vi "ESN_network.vi"(7 "In train phase? (F)":bool, 8 "error in (no error)":errorcluster, 9 "Desired output":dbl[](array[numeric]), 10 "input":dbl[](array[numeric]), 11 "ESN Status":T1) -> (0 "error out":errorcluster, 1 "State collection":dbl[](array[numeric]), 2 "output":dbl[](array[numeric]), 3 "ESN dup":T1)   [LabVIEW 2017]
uses:
  ESN_Network.ctl
  <vilib>/Analysis/Matrix/Datatypes/RealMatrix.ctl
  <vilib>/Analysis/baseanly.llb/A x Vector.vi
  <vilib>/Analysis/NI_AALBase.lvlib
  <vilib>/Analysis/Matrix/NI_Matrix.lvlib
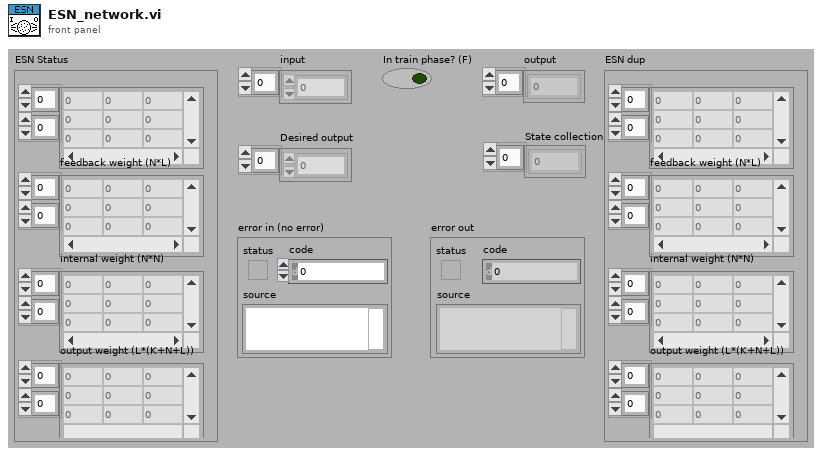
[diagram p1: front panel]
types:
  T1 = typedef "ESN_Network.ctl" = cluster{"output to internal feedback?":bool, "output to output feedback?":bool, "input to output feedforward?":bool, "number of input (K)":i32, "number of internal (N)":i32, "number of output (L)":i32, "input normalization vector":dbl[], "output restore vector":dbl[], "input weight (N*K)":T2, "feedback weight (N*L)":T2, "internal weight (N*N)":T2, "output weight (L*(K+N+L))":T2}
  T2 = typedef "NI_Matrix.lvlib/RealMatrix.ctl" = dbl[][]
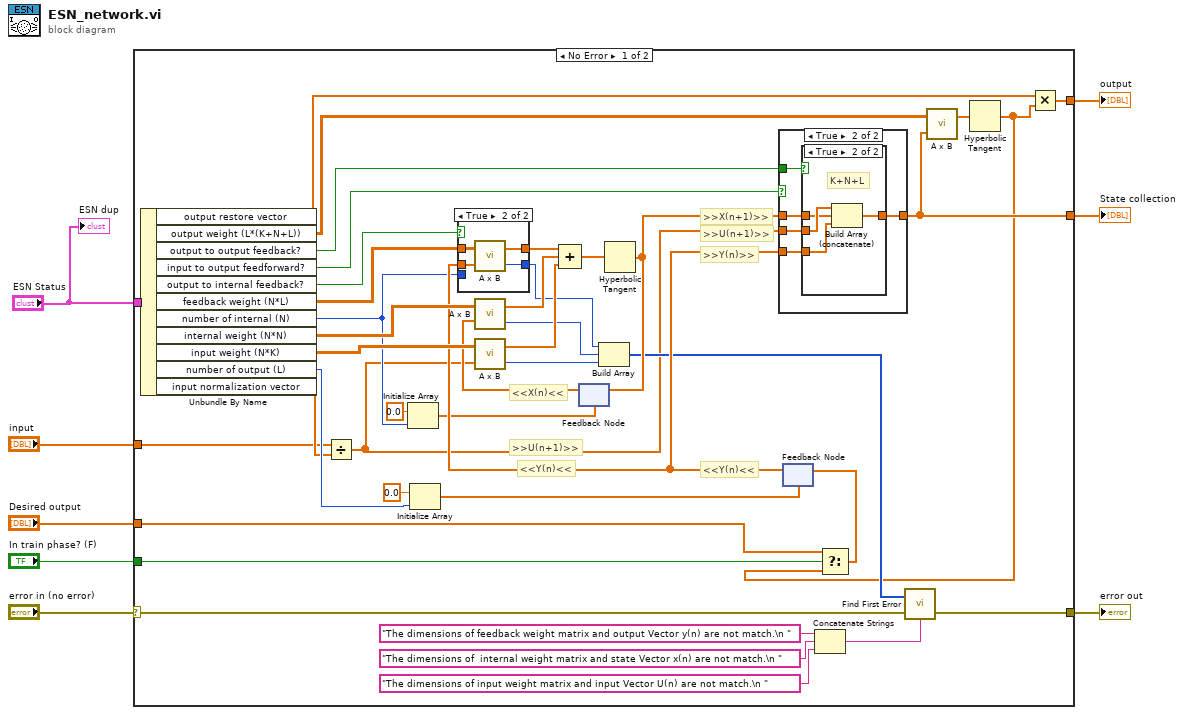
[diagram p0: block diagram]
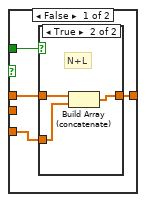
[diagram p2: hidden frame]
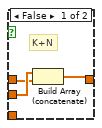
[diagram p4: hidden frame]
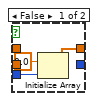
[diagram p5: hidden frame]
diagram:
  n1 = case shown="No Error" "error in (no error)" {
    selector: "error in (no error)" -> [w21 w78]
    tunnel: "ESN Status" -> [w50 _]
    tunnel: "input" -> [w12 _]
    tunnel: [w37 _] -> w7
    tunnel: "In train phase? (F)" -> [w19 _]
    tunnel: "Desired output" -> [w27 _]
    tunnel: [w10 _] -> w4
    tunnel: [w20 w78] -> w2
    frame No Error {
      # ">>Y(n)>>"
      # ">>U(n+1)>>"
      # ">>U(n+1)>>"
      # ">>X(n+1)>>"
      # "<<Y(n)<<"
      # "<<Y(n)<<"
      # "<<X(n)<<"
      n2 = Unbundle By Name(w50) -> ("output restore vector"=w13:dbl[], "output weight (L*(K+N+L))"=w38:T2, "output to output feedback?"=w40:bool, "input to output feedforward?"=w41:bool, "output to internal feedback?"=w43:bool, "feedback weight (N*L)"=w42:T2, "number of internal (N)"=w32:i32, "internal weight (N*N)"=w48:T2, "input weight (N*K)"=w49:T2, "number of output (L)"=w29:i32, "input normalization vector"=w14:dbl[])
      n3 = Divide(x=w12, y=w14) -> (x/y=w9:dbl[])
      n4 = Initialize Array(0.0 ("element"), w32) -> (w31:dbl[])
      n5 = Initialize Array(0.0 ("element"), w29) -> (w28:dbl[])
      n6 = call-poly <vilib>:"A x B.vi"("Vector"=w9, "A"=w49) -> ("error"=w24:i32, "A x Vector"=w45:dbl[])
      n7 = feedback #1(w31) -> (w39:dbl[])
      n8 = call-poly <vilib>:"A x B.vi"("Vector"=w39, "A"=w48) -> ("error"=w25:i32, "A x Vector"=w46:dbl[])
      n9 = feedback #2(w28) -> (w35:dbl[])
      n10 = case shown="True" w43 {
        tunnel: w42 -> [_ w77]
        tunnel: w35 -> [_ w76]
        tunnel: [w71 w75] -> w47
        tunnel: w32 -> [w73 _]
        tunnel: [_ w74] -> w23
        frame False {
          n11 = Initialize Array(0.0 ("element"), w73) -> (w71:dbl[])
        }
        frame True {
          n12 = call-poly <vilib>:"A x B.vi"("Vector"=w76, "A"=w77) -> ("error"=w74:i32, "A x Vector"=w75:dbl[])
        }
      }
      n13 = Compound Arithmetic op=ADD(w47, w46, w45) -> (w44:dbl[])
      n14 = Build Array(w23, w25, w24) -> (w22:i32[])
      n15 = Hyperbolic Tangent(1:w44) -> (0:w34:dbl[])
      n16 = feedback-in #1(w34) -> ()
      n17 = case shown="True" w41 {
        tunnel: w40 -> [w54 w63]
        tunnel: w34 -> [w53 w62]
        tunnel: w9 -> [_ w61]
        tunnel: [w52 w60] -> w37
        tunnel: w35 -> [w51 w59]
        frame False {
          n18 = case shown="True" w54 {
            tunnel: w53 -> [w55 w58]
            tunnel: [w55 w57] -> w52
            tunnel: w51 -> [_ w56]
            frame False {
              # "N"
            }
            frame True {
              # "N+L"
              n19 = Build Array (concatenate)(w58, w56) -> (w57:dbl[])
            }
          }
        }
        frame True {
          n20 = case shown="True" w63 {
            tunnel: w62 -> [w65 w69]
            tunnel: w61 -> [w66 w70]
            tunnel: [w64 w68] -> w60
            tunnel: w59 -> [_ w67]
            frame False {
              # "K+N"
              n21 = Build Array (concatenate)(w66, w65) -> (w64:dbl[])
            }
            frame True {
              # "K+N+L"
              n22 = Build Array (concatenate)(w70, w69, w67) -> (w68:dbl[])
            }
          }
        }
      }
      n23 = Concatenate Strings("The dimensions of feedback weight matrix and output Vector y(n) are not match.\n " ("source messages"), "The dimensions of  internal weight matrix and state Vector x(n) are not match.\n " ("source messages"), "The dimensions of input weight matrix and input Vector U(n) are not match.\n " ("source messages")) -> (w17:string)
      n24 = call <vilib>:"Find First Error.vi"("error in (no error)"=w21, "source messages"=w17, "error codes"=w22) -> ("error out"=w20:errorcluster)  [unwired: 1 in, 1 out]
      n25 = call-poly <vilib>:"A x B.vi"("Vector"=w37, "A"=w38) -> ("A x Vector"=w36:dbl[])  [unwired: 1 out]
      n26 = Hyperbolic Tangent(1:w36) -> (0:w11:dbl[])
      n27 = Select(t=w27, s=w19, f=w11) -> (s? t:f=w26:dbl[])
      n28 = feedback-in #2(w26) -> ()
      n29 = Multiply(x=w13, y=w11) -> (x*y=w10:dbl[])
    }
    frame Error {
    }
  }
  "output" <- w4
  "State collection" <- w7
  "error out" <- w2
  "ESN dup" <- "ESN Status"
